vi "Apply Channel Names.vi"(8 "error in":errorcluster, 11 "PRM in":refnum<class "PRM.lvclass">) -> (0 "error out":errorcluster, 3 "PRM out":refnum<class "PRM.lvclass">)   [LabVIEW 2019, in "PRM.lvlib" / "PRM.lvclass"]
uses:
  Library/PRM.lvclass
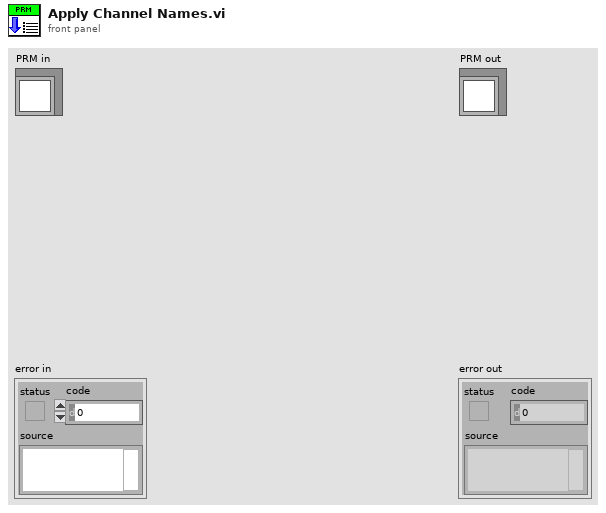
[diagram p1: front panel]
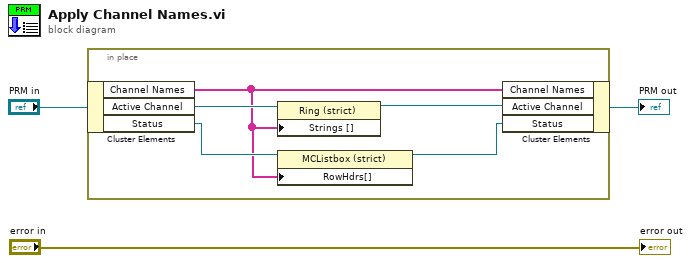
[diagram p0: block diagram]
diagram:
  n1 = in-place {
    n2 = in-place-cluster #1("PRM in") -> ("Channel Names"=w4:string[], "Active Channel"=w8:refnum<vi>, "Status"=w6:refnum<vi>)
    n3 = property class="Ring (strict)"(reference=w8, "Strings []"=w4) -> (reference out=w7:refnum<vi>)  [unwired: 1 in, 1 out]
    n4 = property class="MCListbox (strict)"(reference=w6, "RowHdrs[]"=w4) -> (reference out=w5:refnum<vi>)  [unwired: 1 in, 1 out]
    n5 = in-place-cluster #1("Channel Names"=w4, "Active Channel"=w7, "Status"=w5) -> (→"PRM out":refnum<class "PRM.lvclass">)
  }
  "error out" <- "error in"
